vi "SPIEngineSOM.vi"(7 "NumNodes":u8=1) -> ()   [LabVIEW 2014, in "IO Node Logic Template_SPIBus0.lvlib"]
uses:
  IO Node Logic Template_SPIBus0.lvlib
  <userlib>/_NI SPI IP/FPGA/Controllers/Public/Spi Master Outputs.ctl
  Controls/All Nodes Resources.ctl
  Node/Controls/NodeResources FIFOs.ctl
  <vilib>/Platform/TimedLoop/XDataNode/timing_clust.ctl
  <vilib>/Platform/TimedLoop/XDataNode/nitl_modes.ctl
  <vilib>/Platform/TimedLoop/XDataNode/wakeup.ctl
  <vilib>/rvi/Emulation/niFpgaSctlEmulationGetInTimedLoop.vi
  <vilib>/rvi/Emulation/niFpgaEmulationReportErrorSimple.vi
  <vilib>/rvi/Emulation/niFpgaGetClockAttributes.vi
  <vilib>/rvi/Emulation/niFpgaCriticalErrorInLSC.vi
  <vilib>/Platform/TimedLoop/XDataNode/XDataNode.xnode
  <vilib>/Platform/TimedLoop/XDataNode/XDNodeRunTimeDep.lvlib
  <userlib>/_NI SPI IP/FPGA/Controllers/NI SPI IP FPGA.lvlib
panel:
  out "spi output":T1
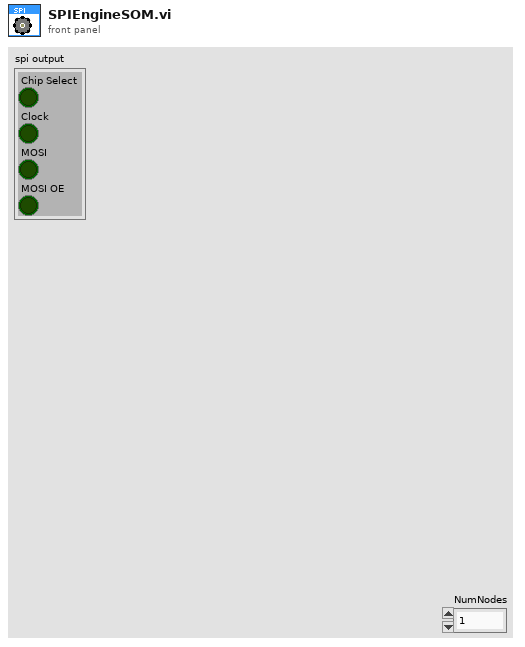
[diagram p1: front panel]
types:
  T1 = typedef "NI SPI IP FPGA.lvlib/Spi Master Outputs.ctl" = cluster{"Chip Select":bool, "Clock":bool, "MOSI":bool, "MOSI OE":bool}
  T2 = typedef "IO Node Logic Template_SPIBus0.lvlib/All Nodes Resources.ctl" = cluster{"FIFOs.Node 0":T3}
  T3 = typedef "IO Node Logic Template_SPIBus0.lvlib/NodeResources FIFOs.ctl" = cluster{"SendCmdFIFO":refnum<k21>, "ReceiveDataFIFO":refnum<k21>}
  T4 = typedef "SPI Digital IO Lines.ctl" = cluster{"SCLK":refnum<k21>, "MISO":refnum<k21>, "MOSI":refnum<k21>, "CS 0":refnum<k21>, "CS 1":refnum<k21>, "CS 2":refnum<k21>, "CS 3":refnum<k21>, "CS 4":refnum<k21>, "CS 5":refnum<k21>}
  T5 = typedef "Internal Data (SPI API).ctl" = cluster{"DLU To SPI Engine Data FIFO":refnum<k21>, "SPI Engine to DLU Data FIFO":refnum<k21>, "Data to SPI Engine (Cache) Register":refnum<k21>, "SPI PHY Settings to SPI Engine (Cahche) Register":refnum<k21>}
  T6 = typedef "XDNodeRunTimeDep.lvlib/timing_clust.ctl" = cluster{"Expected End [f-1]":u64, "Actual End [f-1]":u64, "Finished Late? [f-1]":bool, "Expected End [i-1]":u64, "Actual End [i-1]":u64, "Finished Late? [i-1]":bool, "Expected Start [i]":u64, "Actual Start [i]":u64, "Expected Start [f]":u64, "Actual Start [f]":u64, "Source Name":string, "Structure Name":string, "Period":i64, "Deadline":i64, "Offset":i64, "Start":i64, "Priority":i32, "Timeout":i32, "Mode":T7, "Wakeup Reason":T8, "Error":errorcluster, "Source Type":string, "Secondary Source Type":string, "Global End Time":u64, "Global Start Time":u64, "Frame Duration":u64, "Iteration Duration":u64, "Assigned CPU":i32, "I/O Scan Engine Mode":u32}
  T7 = typedef "XDNodeRunTimeDep.lvlib/nitl_modes.ctl" = enum32{"No Change", "Process missed periods, maintain original phase", "Discard missed periods, maintain original phase", "Process missed periods, ignore original phase", "Discard missed periods, ignore original phase"}
  T8 = typedef "XDNodeRunTimeDep.lvlib/wakeup.ctl" = enum32{"Normal", "Aborted", "Asynchronous wakeup", "Timing source error", "Timed loop error", "Timeout"}
  T9 = typedef "IO Node Logic Template_SPIBus0.lvlib/Node_Command_Sent.ctl" = cluster{"Device ID":u8, "Data":u64, "Command":u8, "Node ID":u8, "Misc":u8}
  T10 = typedef "SPI Response Information.ctl" = cluster{"Data to Node":u64, "Node Id":u16}
  T11 = typedef "NI SPI IP FPGA.lvlib/Spi Master Inputs.ctl" = cluster{"MISO":bool}
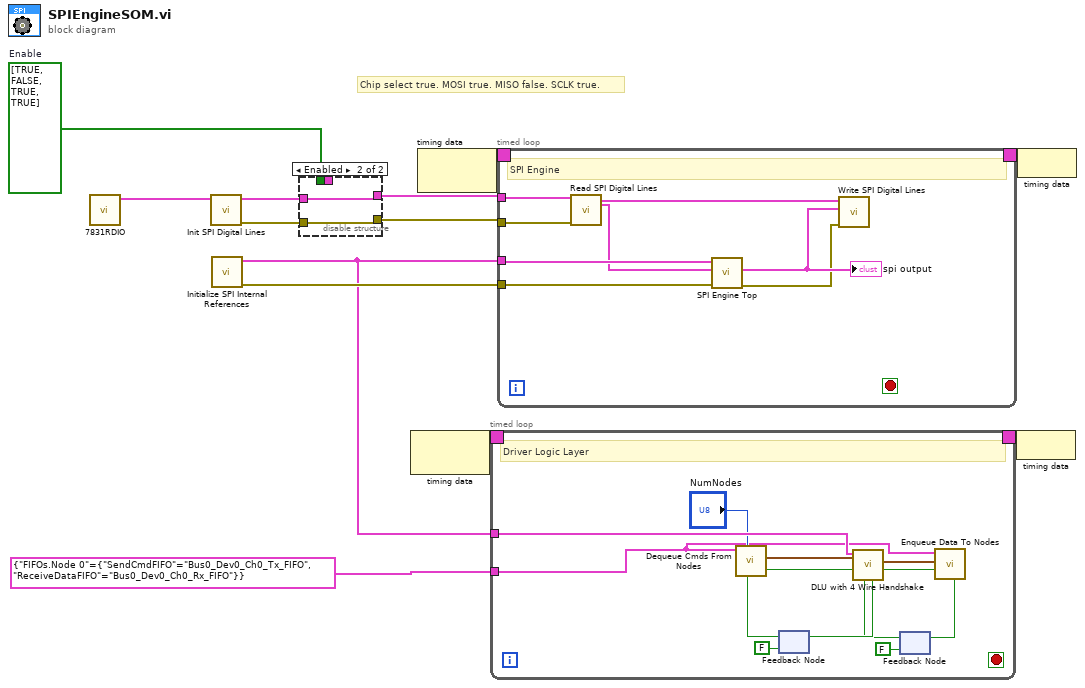
[diagram p0: block diagram]
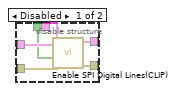
[diagram p2: hidden frame]
diagram:
  w3 = bool[] [TRUE, FALSE, TRUE, TRUE]  # Enable
  # "Chip select true. MOSI true. MISO false. SCLK true."
  n1 = call "7831RDIO.vi"() -> ("SPI DIO Lines"=w1:T4)  [unwired: 11 in]
  n2 = call <vilib>:"Init SPI Digital Lines.vi"("Chip Select DIO Lines"=w1) -> ("error out"=w11:errorcluster, "Chip Select DIO Lines"=w4:T4)  [unwired: 9 in]
  n3 = call <vilib>:"Initialize SPI Internal References.vi"() -> ("error out"=w13:errorcluster, "SPI API References"=w12:T5)  [unwired: 10 in]
  n4 = disable-structure shown="Enabled" {
    disable-tunnel: w11 -> [w19 w20]
    disable-tunnel: [w18 w20] -> w10
    disable-tunnel: [w17 w21] -> w9
    disable-tunnel: _ -> [w16 _]
    disable-tunnel: w4 -> [w15 w21]
    disable-tunnel: w3 -> [w14 _]
    frame Disabled {
      n5 = call <vilib>:"Enable SPI Digital Lines(CLIP).vi"("error in"=w19, "Enable"=w14, "Enable Lines"=w16, "SPI DIO Lines"=w15) -> ("error out"=w18:errorcluster, "Chip Select DIO Lines"=w17:T4)  [unwired: 6 in]
    }
    frame Enabled {
    }
  }
  n6 = node-c288() -> (w6:T6)  [unwired: 1 in]
  n7 = node-c288() -> (w8:T6)  [unwired: 1 in]
  n8 = timed-loop {
    tunnel: w12 -> [w25]
    timing: w6 -> [_]
    timing-out: [_] -> w5
    tunnel: T2 {"FIFOs.Node 0"={"SendCmdFIFO"="Bus0_Dev0_Ch0_Tx_FIFO", "ReceiveDataFIFO"="Bus0_Dev0_Ch0_Rx_FIFO"}} ("Communication FIFOs") -> [w22]
    stop <- _ stop-if-true
    # "Driver Logic Layer"
    n9 = feedback #1(FALSE ("Ready For Input?")) -> (w32:bool)
    n10 = call "Dequeue Cmds From Nodes.vi"("Ready For Output?"=w32, "NumNodes"="NumNodes", "Communication FIFOs"=w22) -> ("Cmd Received Valid"=w30:bool, "Cmd Received"=w29:T9)  [unwired: 5 in, 2 out]
    n11 = feedback #2(FALSE ("Ready for Input")) -> (w27:bool)
    n12 = call "DLU with 4 Wire Handshake.vi"("ready for output"=w27, "Input Valid"=w30, "Input Data"=w29, "Private Data In"=w25) -> ("Output Valid"=w34:bool, "Output Data"=w24:T10, "ready for Input"=w31:bool)  [unwired: 5 in]
    n13 = feedback-in #1(w31) -> ()
    n14 = call "Enqueue Data To Nodes.vi"("Input Valid"=w34, "Input Data"=w24, "Communication FIFOs"=w22) -> ("Ready for Input"=w28:bool)  [unwired: 6 in, 2 out]
    n15 = feedback-in #2(w28) -> ()
  }
  n16 = timed-loop {
    tunnel: w12 -> [w44]
    tunnel: w13 -> [w43]
    tunnel: w9 -> [w42]
    tunnel: w10 -> [w41]
    timing: w8 -> [_]
    timing-out: [_] -> w7
    stop <- _ stop-if-true
    # "SPI Engine"
    n17 = call <vilib>:"Read SPI Digital Lines.vi"("Chip Select DIO Lines"=w42, "error in"=w41) -> ("Chip Select DIO Lines Out"=w40:T4, "SPI Read Data"=w38:T11)  [unwired: 11 in, 1 out]
    n18 = call <vilib>:"SPI Engine Top.vi"("error in"=w43, "SPI Read Data"=w38, "SPI API References"=w44) -> ("error out"=w37:errorcluster, "SPI DIO Output"=w39:T1)  [unwired: 5 in, 2 out]
    "spi output" <- w39
    n19 = call <vilib>:"Write SPI Digital Lines.vi"("error in"=w37, "spi output"=w39, "Chip Select DIO Lines"=w40) -> ()  [unwired: 7 in, 2 out]
  }
  n20 = node-c288(w5) -> ()
  n21 = node-c288(w7) -> ()
